vi "Stop Chassis.vi"(8 "error in (no error)":errorcluster, 10 "final error code":i32, 11 "HS Only in":refnum<class "HS Only.lvclass">) -> (0 "error out":errorcluster, 2 "Max Read Time (ms)":i32, 3 "HS Only out":refnum<class "HS Only.lvclass">)   [LabVIEW 2018, in "Data Acquisition.lvlib" / "HS Only.lvclass"]
uses:
  HS Only.lvclass
  C:/Users/Jeff Tipps/Documents/DAQMan/source/Classes/Data Acquisition/Class Chassis Tasks/Chassis Tasks.lvclass
  Class Chassis Tasks/Chassis Tasks.lvclass/Chassis Tasks.ctl
  <vilib>/ActorFramework/Stop Msg/Stop Msg.lvclass/Stop Msg.ctl
  <vilib>/ActorFramework/Message Enqueuer/Message Enqueuer.lvclass/Message Enqueuer.ctl
  Class Chassis Tasks/Read HS DAQ Task.vi
  Class Chassis Tasks/Read HS ActorQ.vi
  <vilib>/ActorFramework/Stop Msg/Send Emergency Stop.vi
  <vilib>/ActorFramework/Stop Msg/Send Normal Stop.vi
  <vilib>/ActorFramework/Message Enqueuer/Enqueue Critical.vi
  <vilib>/ActorFramework/Message Enqueuer/Enqueue.vi
  <vilib>/ActorFramework/Stop Msg/Stop Msg.lvclass
  C:/Program Files (x86)/National Instruments/LabVIEW 2018/vi.lib/ActorFramework/Message/Message.lvclass
  <vilib>/ActorFramework/Message Priority Queue/Priority Enqueue.vi
  Class DAQ Task/DAQ Task.lvclass
  <vilib>/ActorFramework/Message Enqueuer/Message Enqueuer.lvclass
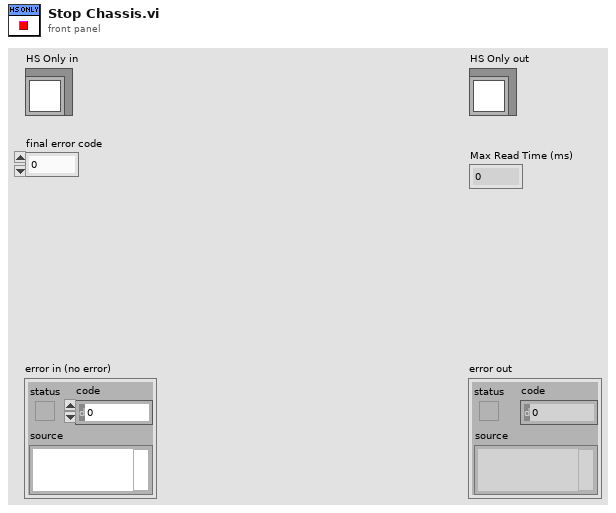
[diagram p1: front panel]
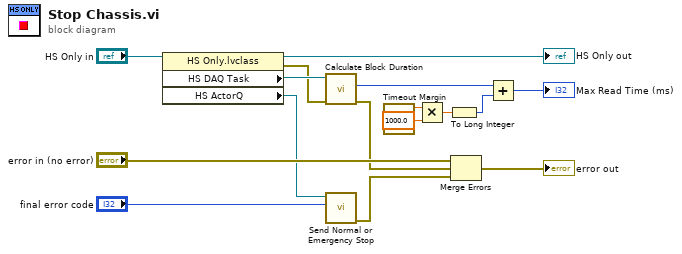
[diagram p0: block diagram]
diagram:
  n1 = property class="HS Only.lvclass"(reference="HS Only in") -> (reference out=→"HS Only out":refnum<class "HS Only.lvclass">, error out=w8:errorcluster, "HS DAQ Task"=w9:refnum<class "DAQ Task.lvclass">, "HS ActorQ"=w10:refnum<class "Message Enqueuer.lvclass">)  [unwired: 1 in]
  n2 = call "Calculate Block Duration.vi"("error in (no error)"=w8, "DAQ Task in"=w9) -> ("error out"=w7:errorcluster, "Block Duration (ms)"=w3:i32)  [unwired: 7 in, 1 out]
  n3 = call <vilib>:"Send Normal or Emergency Stop.vi"("final error code"="final error code", "Message Enqueuer"=w10) -> ("error out"=w14:errorcluster)  [unwired: 9 in]
  n4 = call "Timeout Margin.vi"() -> ("y"=w6:dbl)  [unwired: 11 in]
  n5 = Multiply(x=w6, y=1000.0) -> (x*y=w4:dbl)
  n6 = To Long Integer(number=w4) -> (32bit integer=w2:i32)
  n7 = Merge Errors("error in (no error)", w7, w14) -> (→"error out":errorcluster)
  n8 = Add(x=w3, y=w2) -> (x+y=→"Max Read Time (ms)":i32)
